vi "Set Trigger Slope.vi"(8 "error in (no error)":errorcluster, 10 "j (0)":enum16{"Rise", "Fall"}(ring), 11 "VISA resource name":refnum<visa-resource-name>) -> (0 "error out":errorcluster, 3 "VISA resource name out":refnum<visa-resource-name>)   [LabVIEW 2015, in "SR400.lvlib"]
doc: "TS { j }\nIf j = 1, the TS command sets the gate trigger\nslope to FALL or negative. If j = 0, the gate trigger\nslope is set to RISE or positive. If j is absent, the\ngate trigger slope is returned."
uses:
  SR400.lvlib
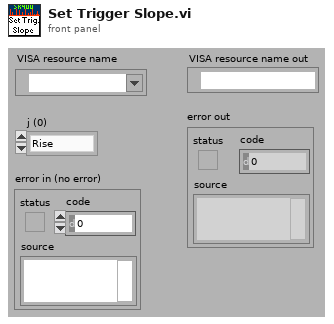
[diagram p1: front panel]
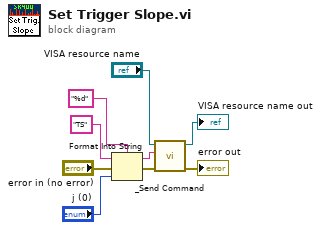
[diagram p0: block diagram]
diagram:
  n1 = Format Into String(format string="%d", initial string="TS" ("command"), error in="error in (no error)", "j (0)") -> (resulting string=w4:string, error out=w3:errorcluster)
  n2 = call "_Send Command.vi"("error in (no error)"=w3, "Command"=w4, "VISA resource name"="VISA resource name") -> ("error out"=→"error out":errorcluster, "VISA resource name out"=→"VISA resource name out":refnum<visa-resource-name>)  [unwired: 1 in, 6 out]
